vi "boolean to channel list.vi"(11 "target channels":bool[](array[boolean])) -> (2 "open":string, 3 "close":string)   [LabVIEW 2018]
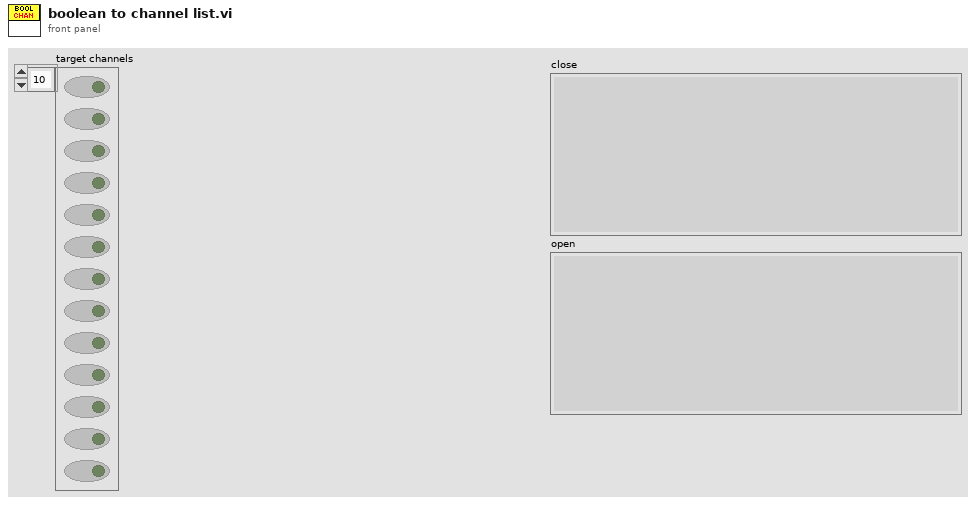
[diagram p1: front panel]
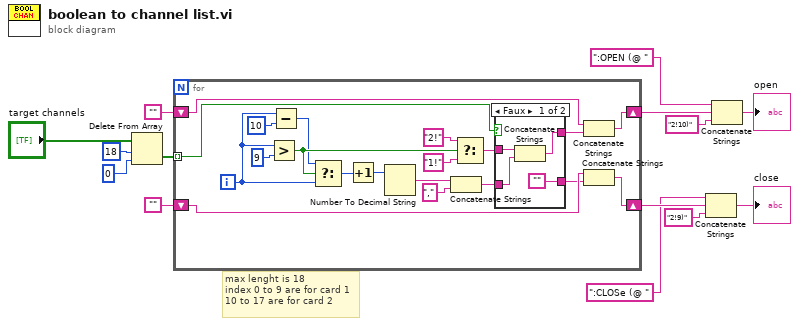
[diagram p0: block diagram]
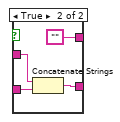
[diagram p2: hidden frame]
diagram:
  # "max lenght is 18\nindex 0 to 9 are for card 1\n10 to 17 are for card 2"
  n1 = Delete From Array(array="target channels", length=18 ("longueur"), index=0 ("indice")) -> (deleted portion=w7:bool[])  [unwired: 1 out]
  n2 = for {
    tunnel: w7 -> [w21] mode=indexing
    shift-right: [w34] -> w14
    shift-left: "" -> [w33]
    shift-right: [w16] -> w2
    shift-left: "" -> [w17]
    i -> [w24]
    n3 = Greater?(x=w24, y=9) -> (0:w27:bool)
    n4 = Subtract(x=w24, y=10) -> (x-y=w25:i32)
    n5 = Select(t=w25, s=w27, f=w24) -> (s? t:f=w23:i32)
    n6 = Increment(x=w23) -> (x+1=w22:i32)
    n7 = Number To Decimal String(number=w22) -> (decimal integer string=w32:string)  [unwired: 1 in]
    n8 = Concatenate Strings(w32, "," ("chaîne")) -> (w19:string)
    n9 = Select(t="2!" ("chaîne"), s=w27, f="1!" ("chaîne")) -> (s? t:f=w20:string)
    n10 = case shown="Faux" w21 {
      tunnel: w20 -> [w37 w41]
      tunnel: w19 -> [w35 w40]
      tunnel: ["" w39] -> w18
      tunnel: [w36 ""] -> w15
      frame False {
        n11 = Concatenate Strings(w37, w35) -> (w36:string)
      }
      frame True {
        n12 = Concatenate Strings(w41, w40) -> (w39:string)
      }
    }
    n13 = Concatenate Strings(w17, w15) -> (w16:string)
    n14 = Concatenate Strings(w33, w18) -> (w34:string)
  }
  n15 = Concatenate Strings(":CLOSe (@ " ("chaîne"), w14, "2!9)" ("chaîne")) -> (→"close":string)
  n16 = Concatenate Strings(":OPEN (@ " ("chaîne"), w2, "2!10)" ("chaîne")) -> (→"open":string)
